vi "Changer.vi"(0 "toChanger":T1(array[cluster]), 1 "out":i8[](array[numeric]), 2 "in":i8[](array[numeric])) -> ()   [LabVIEW 2009]
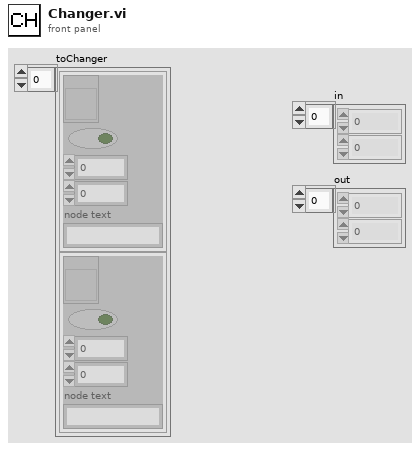
[diagram p1: front panel]
types:
  T1 = cluster{refnum<vi>, bool, i32, i32, "node text":string}[]
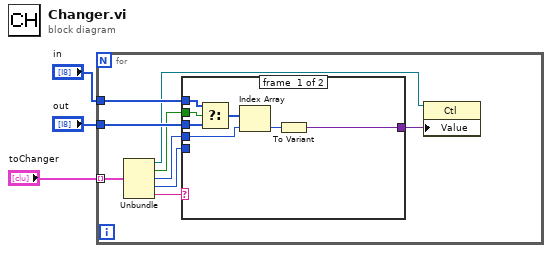
[diagram p0: block diagram]
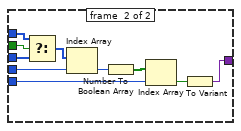
[diagram p2: hidden frame]
diagram:
  n1 = for {
    tunnel: "out" -> [w12]
    tunnel: "toChanger" -> [w11] mode=indexing
    tunnel: "in" -> [w9]
    n2 = Unbundle(w11) -> (w5:refnum<vi>, w8:bool, w7:i32, w10:i32, "node text"=w6:string)
    n3 = case shown="\"Boolean\"" w6 {
      tunnel: w12 -> [w19 w28]
      tunnel: [w17 w24] -> w4
      tunnel: w10 -> [_ w23]
      tunnel: w9 -> [w16 w22]
      tunnel: w8 -> [w15 w21]
      tunnel: w7 -> [w14 w20]
      frame #0 {
        n4 = Select(t=w16, s=w15, f=w19) -> (s? t:f=w18:i8[])
        n5 = Index Array(array=w18, index=w14) -> (element=w13:i8)
        n6 = To Variant(anything=w13) -> (Variant=w17:variant)
      }
      frame #1 {
        n7 = Select(t=w22, s=w21, f=w28) -> (s? t:f=w27:i8[])
        n8 = Index Array(array=w27, index=w20) -> (element=w26:i8)
        n9 = Number To Boolean Array(number=w26) -> (Boolean array=w29:bool[])
        n10 = Index Array(array=w29, index=w23) -> (element=w25:bool)
        n11 = To Variant(anything=w25) -> (Variant=w24:variant)
      }
    }
    n12 = property on="Property Node" class="Ctl"(reference=w5, "Value"=w4) -> ()  [unwired: 1 in, 2 out]
  }
